vi "3.2.vi"() -> ()   [LabVIEW 2020]
uses:
  <vilib>/numeric/Random Number (Range) I64.vi
  <vilib>/numeric/sub_Random U32.vi
  <vilib>/measure/NI_MABase.lvlib
panel:
  in  "stop":bool
  out "AMPLITUD MAXIMA":dbl
  out "Grafica":waveform(dbl)[](graph)
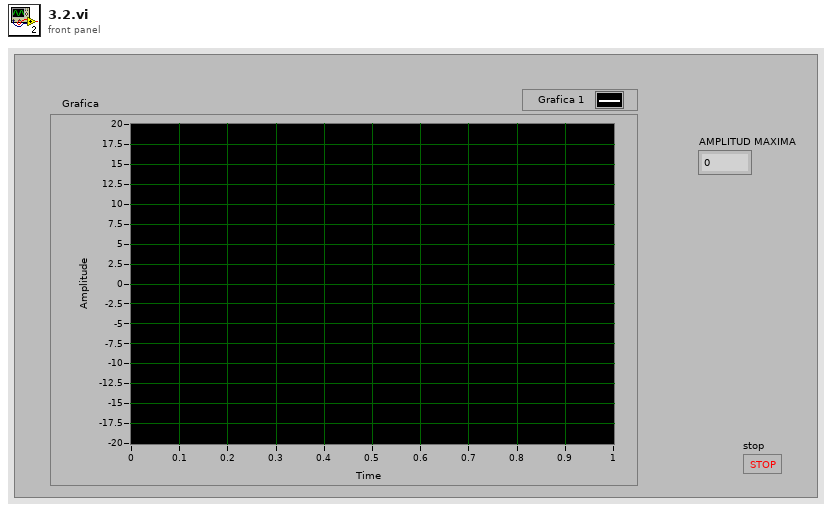
[diagram p1: front panel]
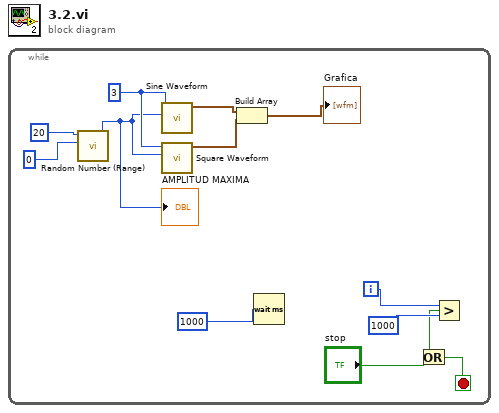
[diagram p0: block diagram]
diagram:
  n1 = while {
    i -> [w10]
    stop <- w11 stop-if-true
    w6 = 3
    n2 = call-poly <vilib>:"Random Number (Range).vi"("lower bound (-100)"=0, "upper bound (100)"=20) -> ("number"=w2:i64)  [unwired: 9 in]
    "AMPLITUD MAXIMA" <- w2
    n3 = call <vilib>:"Sine Waveform.vi"("amplitude"=w2, "frequency"=w6) -> ("signal out"=w5:waveform(dbl))  [unwired: 8 in, 1 out]
    n4 = call <vilib>:"Square Waveform.vi"("amplitude"=w2, "frequency"=w6) -> ("signal out"=w4:waveform(dbl))  [unwired: 8 in, 1 out]
    n5 = Build Array(w5, w4) -> (→"Grafica":waveform(dbl)[])
    n6 = Wait (ms)(milliseconds to wait=1000) -> ()  [unwired: 1 out]
    n7 = Greater?(x=w10, y=1000) -> (0:w8:bool)
    n8 = Or(x=w8, y="stop") -> (x .or. y?=w11:bool)
  }
